vi "Write Submodule EOL.vi"(8 "error in (no error)":errorcluster, 10 "Submodule EOL":T1={"PLC Folder Names"=[], "Timeout Connect OPC"=0.0, "Connect OPC Trial"=0, "PLC URL"="", "Digitial IO"="", "HiPOT"="", "ACIR with Switch"="", "DMM with Switch"="", "Ignition Folder Names"=[], "Ignition URL"="", "Test Name"="Battery Submodule EOL"} {"Timeout Connect OPC" format="%#_f"}, 11 "Submodule EOL configuration":refnum<class "Submodule EOL configuration.lvclass">) -> (0 "error out":errorcluster, 3 "Submodule EOL configuration out":refnum<class "Submodule EOL configuration.lvclass">)   [LabVIEW 2025, in "Submodule EOL.lvlib" / "Submodule EOL configuration.lvclass"]
uses:
  Submodule EOL configuration.lvclass
  Submodule EOL.ctl
  Submodule EOL configuration.lvclass/Submodule EOL configuration.ctl
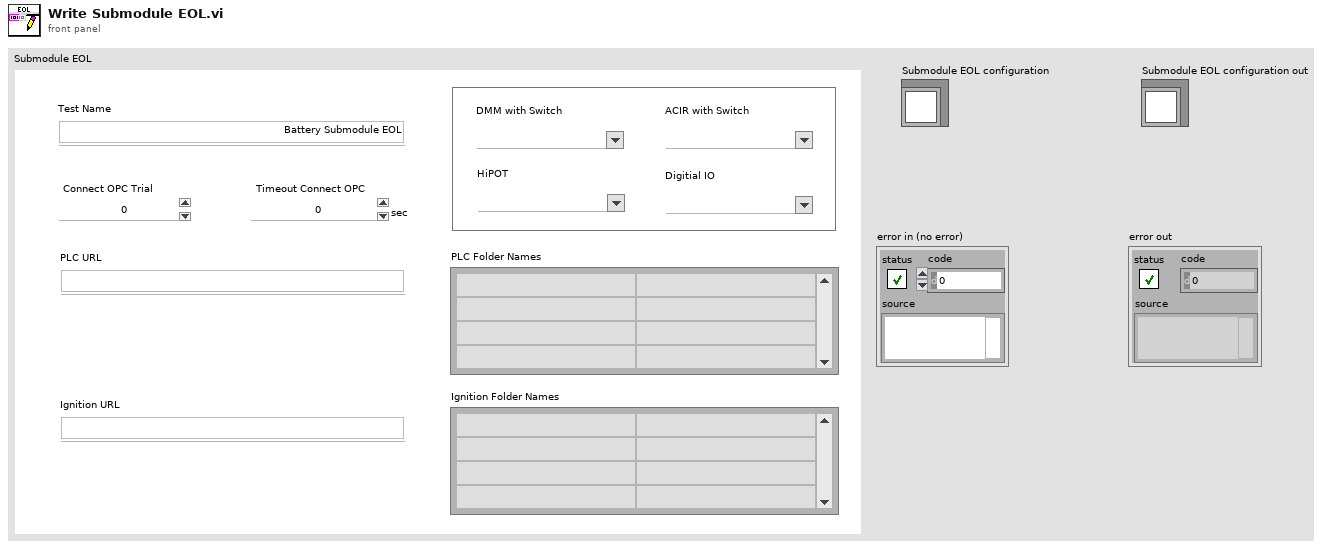
[diagram p1: front panel]
types:
  T1 = typedef "Submodule EOL.lvlib/Submodule EOL configuration.lvclass/Submodule EOL.ctl" = cluster{"PLC Folder Names":string[][], "Timeout Connect OPC":dbl, "Connect OPC Trial":u32, "PLC URL":string, "Digitial IO":string, "HiPOT":string, "ACIR with Switch":string, "DMM with Switch":string, "Ignition Folder Names":string[][], "Ignition URL":string, "Test Name":string}
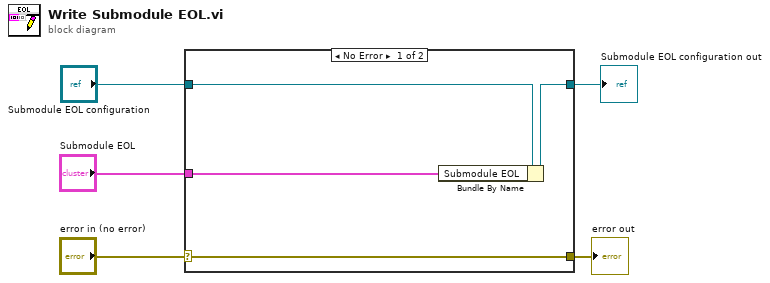
[diagram p0: block diagram]
diagram:
  n1 = case shown="No Error" "error in (no error)" {
    selector: "error in (no error)" -> [w9 w10]
    tunnel: [w9 w10] -> w4
    tunnel: [w7 w11] -> w1
    tunnel: "Submodule EOL configuration" -> [w8 w11]
    tunnel: "Submodule EOL" -> [w6 _]
    frame No Error {
      n2 = Bundle By Name(cluster=w8, "Submodule EOL"=w6) -> (w7:refnum<class "Submodule EOL configuration.lvclass">)
    }
    frame Error {
    }
  }
  "error out" <- w4
  "Submodule EOL configuration out" <- w1
